vi "MT Measure Rho.vi"(0 "received complex waveform":cluster{"t0":dbl, "dt":dbl, "Y":cdb[]} {"Y" format="%.3f"; "dt" format="%^.2e"; "t0" format="%.4f"}, 5 "ideal complex waveform":cluster{"t0":dbl, "dt":dbl, "Y":cdb[]} {"Y" format="%.3f"; "dt" format="%^.2e"; "t0" format="%.4f"}, 11 "error in (no error)":errorcluster) -> (4 "rho":dbl format="%.4f", 15 "error out":errorcluster)   [LabVIEW 2020, in "niDMT.lvlib"]
doc: "Calculates rho given an acquired and ideal waveform. Rho is a measure of correlation between the <B>measured complex waveform</B> and the <B>ideal complex waveform</B>. To generate the ideal waveform, use the digital modulation VIs with the same system parameters given to the digital demodulation VIs, and then modulate the <B>output bit stream</B> returned by the demodulation VI."
uses:
  <vilib>/addons/Modulation/niDMT.lvlib
  <vilib>/addons/Modulation/niAMT.lvlib
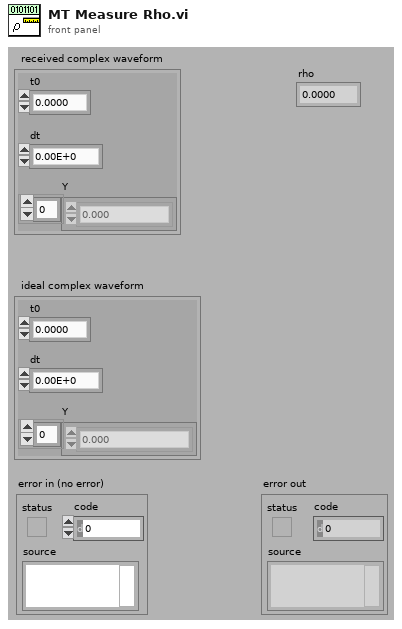
[diagram p1: front panel]
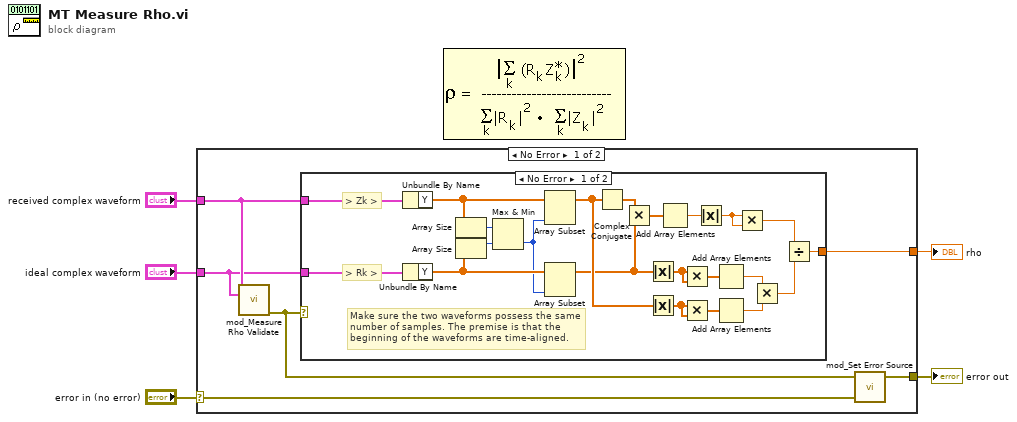
[diagram p0: block diagram]
diagram:
  n1 = case shown="No Error" "error in (no error)" {
    selector: "error in (no error)" -> [w10 w34]
    tunnel: [w11 _] -> w5
    tunnel: "ideal complex waveform" -> [w8 _]
    tunnel: "received complex waveform" -> [w9 _]
    tunnel: [w6 w34] -> w1
    frame No Error {
      n2 = call <vilib>:"mod_Measure Rho Validate.vi"("Received Complex Waveform"=w9, "Ideal Complex Waveform"=w8) -> ("error out"=w7:errorcluster)  [unwired: 13 out]
      n3 = case shown="No Error" w7 {
        tunnel: [w21 _] -> w11
        tunnel: w8 -> [w20 _]
        tunnel: w9 -> [w19 _]
        frame No Error {
          # "Make sure the two waveforms possess the same number of samples. The premise is that the beginning of the waveforms are time-aligned."
          # "> Rk >"
          # "> Zk >"
          n4 = Unbundle By Name(w19) -> ("Y"=w15:cdb[])
          n5 = Unbundle By Name(w20) -> ("Y"=w14:cdb[])
          n6 = Array Size(array=w15) -> (size(s)=w17:i32)
          n7 = Array Size(array=w14) -> (size(s)=w18:i32)
          n8 = Max & Min(x=w17, y=w18) -> (min(x,y)=w12:i32)  [unwired: 1 out]
          n9 = Array Subset(array=w15, length=w12) -> (w16:cdb[])  [unwired: 1 in]
          n10 = Array Subset(array=w14, length=w12) -> (w13:cdb[])  [unwired: 1 in]
          n11 = Complex Conjugate(1:w16) -> (0:w33:cdb[])
          n12 = Multiply(x=w33, y=w13) -> (x*y=w32:cdb[])
          n13 = Absolute Value(x=w13) -> (abs(x)=w26:dbl[])
          n14 = Absolute Value(x=w16) -> (abs(x)=w27:dbl[])
          n15 = Add Array Elements(numeric array=w32) -> (sum=w31:cdb)
          n16 = Multiply(x=w26, y=w26) -> (x*y=w29:dbl[])
          n17 = Multiply(x=w27, y=w27) -> (x*y=w28:dbl[])
          n18 = Absolute Value(x=w31) -> (abs(x)=w30:dbl)
          n19 = Add Array Elements(numeric array=w29) -> (sum=w25:dbl)
          n20 = Add Array Elements(numeric array=w28) -> (sum=w23:dbl)
          n21 = Multiply(x=w30, y=w30) -> (x*y=w24:dbl)
          n22 = Multiply(x=w25, y=w23) -> (x*y=w22:dbl)
          n23 = Divide(x=w24, y=w22) -> (x/y=w21:dbl)
        }
        frame Error {
        }
      }
      n24 = call <vilib>:"mod_Set Error Source.vi"("initial error in (no error)"=w10, "final error in (no error)"=w7) -> ("error out"=w6:errorcluster)  [unwired: 3 out]
    }
    frame Error {
    }
  }
  "rho" <- w5
  "error out" <- w1
